vi "Stream_data.vi"(7 "VISA resource name in":refnum<visa-resource-name>, 8 "error in (no error)":errorcluster, 9 "Notifier error in":errorcluster, 10 "Play / Pause":bool, 11 "Notifier in":refnum<notifier>) -> (0 "VISA error out":errorcluster, 1 "Notifier error out":errorcluster, 2 "read buffer":string, 3 "VISA Refnum out":refnum<visa-resource-name>, 4 "Current time":timestamp)   [LabVIEW 2016]
uses:
  <vilib>/Instr/_visa.llb/VISA Flush IO Buffer Mask.ctl
  Globaltracker.vi
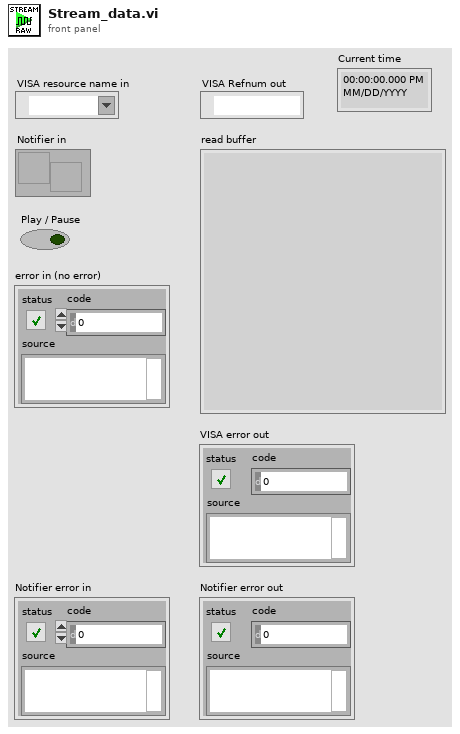
[diagram p1: front panel]
types:
  T1 = typedef "VISA Flush IO Buffer Mask.ctl" = u16
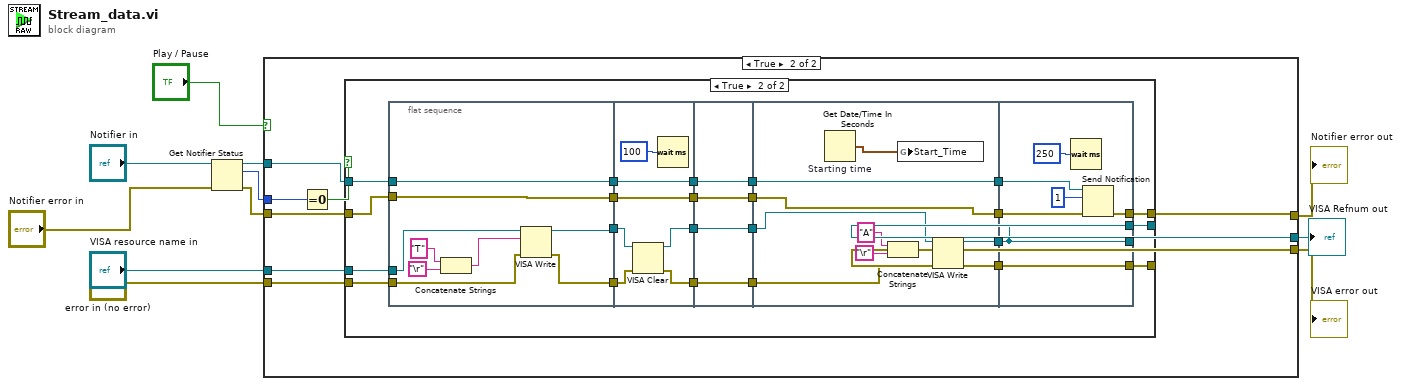
[diagram p0: block diagram]
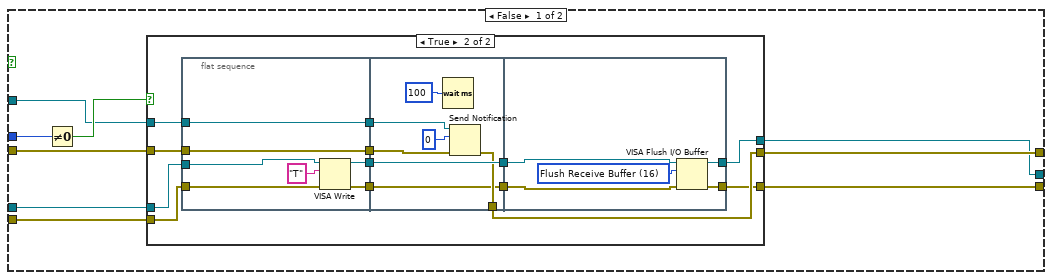
[diagram p2: hidden frame]
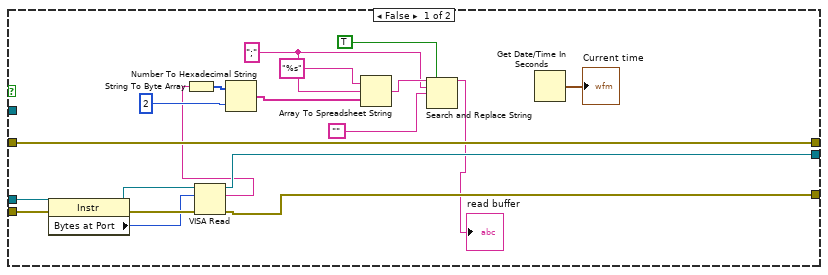
[diagram p4: hidden frame]
diagram:
  n1 = Get Notifier Status(notifier="Notifier in", error in (no error)="Notifier error in") -> (notifier out=w8:refnum<notifier>, current notification=w11:i32, error out=w9:errorcluster)  [unwired: 2 out]
  n2 = case shown="True" "Play / Pause" {
    tunnel: [w12 w56] -> w1
    tunnel: [w13 w57] -> w2
    tunnel: w11 -> [w20 w63]
    tunnel: "error in (no error)" -> [w18 w62]
    tunnel: "VISA resource name in" -> [w17 w61]
    tunnel: w8 -> [w16 w60]
    tunnel: w9 -> [w15 w59]
    tunnel: [w14 w58] -> w10
    frame False {
      n3 = Not Equal To 0?(x=w20) -> (x != 0?=w19:bool)
      n4 = case shown="True" w19 {
        tunnel: w18 -> [w23 w32]
        tunnel: w17 -> [w22 w31]
        tunnel: w16 -> [_ w30]
        tunnel: w15 -> [w21 w29]
        tunnel: [w21 w28] -> w14
        tunnel: [w22 w27] -> w13
        tunnel: [w23 w26] -> w12
        frame False {
        }
        frame True {
          n5 = flat-sequence {
            tunnel: w31 -> [w43]
            tunnel: w32 -> [w42]
            tunnel: [w41] -> w36
            tunnel: [w40] -> w35
            tunnel: [w39] -> w34
            tunnel: w30 -> [w39]
            tunnel: [w38] -> w33
            tunnel: w29 -> [w38]
            tunnel: w36 -> [w49]
            tunnel: w35 -> [w44]
            tunnel: [w48] -> w28
            tunnel: w34 -> [w47]
            tunnel: w33 -> [w46]
            tunnel: [w49] -> w25
            tunnel: [w44] -> w24
            tunnel: [w55] -> w26
            tunnel: [w52] -> w27
            tunnel: w25 -> [w53]
            tunnel: w24 -> [w54]
            frame #0 {
              n6 = VISA Write(VISA resource name=w43, write buffer="T", error in (no error)=w42) -> (VISA resource name out=w41:refnum<visa-resource-name>, error out=w40:errorcluster)  [unwired: 1 out]
            }
            frame #1 {
              n7 = Wait (ms)(milliseconds to wait=u32 100) -> ()  [unwired: 1 out]
              n8 = Send Notification(notification=0, notifier=w47, error in (no error)=w46) -> (error out=w48:errorcluster)  [unwired: 1 out]
            }
            frame #2 {
              w51 = T1 16 items=["Flush Receive Buffer"=16, "Write Transmit Buffer to Device"=32, "Flush Receive Buffer (No I/O)"=64, "Flush Transmit Buffer"=128] ("Mask")
              n9 = VISA Flush I/O Buffer(VISA resource name=w53, mask (16)=w51, error in (no error)=w54) -> (VISA resource name out=w52:refnum<visa-resource-name>, error out=w55:errorcluster)
            }
          }
        }
      }
    }
    frame True {
      n10 = Equal To 0?(x=w63) -> (x = 0?=w64:bool)
      n11 = case shown="True" w64 {
        tunnel: w62 -> [w83 w102]
        tunnel: w61 -> [w82 w101]
        tunnel: w60 -> [_ w100]
        tunnel: w59 -> [w76 w99]
        tunnel: [w76 w98] -> w58
        tunnel: [w78 w97] -> w57
        tunnel: [w77 w96] -> w56
        frame False {
          w70 = ";" ("delimiter (Tab)")
          n12 = property class="Instr"(reference=w82, error in=w83) -> (reference out=w81:refnum<visa-resource-name>, error out=w80:errorcluster, "Bytes at Port"=w79:u32)
          n13 = VISA Read(VISA resource name=w81, byte count=w79, error in (no error)=w80) -> (VISA resource name out=w78:refnum<visa-resource-name>, read buffer=w68:string, error out=w77:errorcluster)  [unwired: 1 out]
          n14 = String To Byte Array(string=w68) -> (unsigned byte array=w75:u8[])
          n15 = Number To Hexadecimal String(1:i16 2 ("width (-)"), 2:w75) -> (0:w73:string[])
          n16 = Array To Spreadsheet String(delimiter (Tab)=w70, array=w73, 3:"%s" ("format string")) -> (spreadsheet string=w71:string)
          n17 = Search and Replace String(replace all?=TRUE ("replace all? (F)"), input string=w71, search string=w70, replace string="") -> (result string=→"read buffer":string)  [unwired: 4 in, 3 out]
          n18 = Get Date/Time In Seconds ("Current time")() -> (seconds since 1Jan1904=→"Current time":timestamp)
        }
        frame True {
          n19 = flat-sequence {
            tunnel: w102 -> [w111]
            tunnel: w101 -> [w112]
            tunnel: w99 -> [w114]
            tunnel: w100 -> [w115]
            tunnel: [w115] -> w95
            tunnel: [w114] -> w94
            tunnel: [w113] -> w93
            tunnel: [w110] -> w92
            tunnel: w95 -> [w122]
            tunnel: [w122] -> w91
            tunnel: w94 -> [w121]
            tunnel: [w121] -> w89
            tunnel: w93 -> [w117]
            tunnel: [w116] -> w87
            tunnel: w92 -> [w119]
            tunnel: [w118] -> w85
            tunnel: w91 -> [w126]
            tunnel: [w126] -> w90
            tunnel: w89 -> [w125]
            tunnel: [w125] -> w88
            tunnel: w87 -> [w124]
            tunnel: [w124] -> w86
            tunnel: w85 -> [w123]
            tunnel: [w123] -> w84
            tunnel: [w133] -> w106
            tunnel: [w132] -> w105
            tunnel: [w129] -> w104
            tunnel: [w128] -> w103
            tunnel: w90 -> [w133]
            tunnel: w88 -> [w132]
            tunnel: w86 -> [w131]
            tunnel: w84 -> [w130]
            tunnel: w106 -> [w142]
            tunnel: w105 -> [w141]
            tunnel: [w139] -> w98
            tunnel: [w138] -> w96
            tunnel: w104 -> [w138]
            tunnel: [w137] -> _
            tunnel: w103 -> [w137]
            tunnel: [w137] -> w97
            frame #0 {
              n20 = Concatenate Strings("T" ("write buffer"), "\r") -> (w107:string)
              n21 = VISA Write(VISA resource name=w112, write buffer=w107, error in (no error)=w111) -> (VISA resource name out=w113:refnum<visa-resource-name>, error out=w110:errorcluster)  [unwired: 1 out]
            }
            frame #1 {
              n22 = VISA Clear(VISA resource name=w117, error in (no error)=w119) -> (VISA resource name out=w116:refnum<visa-resource-name>, error out=w118:errorcluster)
              n23 = Wait (ms)(milliseconds to wait=u32 100) -> ()  [unwired: 1 out]
            }
            frame #2 {
            }
            frame #3 {
              n24 = Get Date/Time In Seconds "Starting time"() -> (seconds since 1Jan1904=w127:timestamp)
              n25 = Concatenate Strings("A" ("write buffer"), "\r") -> (w134:string)
              n26 = global write "Globaltracker.vi" "Start_Time"(w127) -> ()
              n27 = VISA Write(VISA resource name=w131, write buffer=w134, error in (no error)=w130) -> (VISA resource name out=w128:refnum<visa-resource-name>, error out=w129:errorcluster)  [unwired: 1 out]
            }
            frame #4 {
              n28 = Wait (ms)(milliseconds to wait=u32 250) -> ()  [unwired: 1 out]
              n29 = Send Notification(notification=1, notifier=w142, error in (no error)=w141) -> (error out=w139:errorcluster)  [unwired: 1 out]
            }
          }
        }
      }
    }
  }
  "Notifier error out" <- w10
  "VISA Refnum out" <- w2
  "VISA error out" <- w1
